vi "Get Channel Array Variables.vi"(8 "error in (no error)":errorcluster, 11 "LabVIEW Web Service Request":refnum<class "Web Request.lvclass">) -> (0 "error out":errorcluster, 3 "LabVIEW Web Service Request out":refnum<class "Web Request.lvclass">)   [LabVIEW 2018]
doc: "This VI sets all of the ESP variables for a single contact so it can be output from an ESP script."
uses:
  <vilib>/wsapi/Web Request.lvclass
  CAEN globals.vi
  <vilib>/wsapi/class/subVIs/Set Many String ESP Variables.vi
  <vilib>/wsapi/class/subVIs/Set Integer ESP Variable.vi
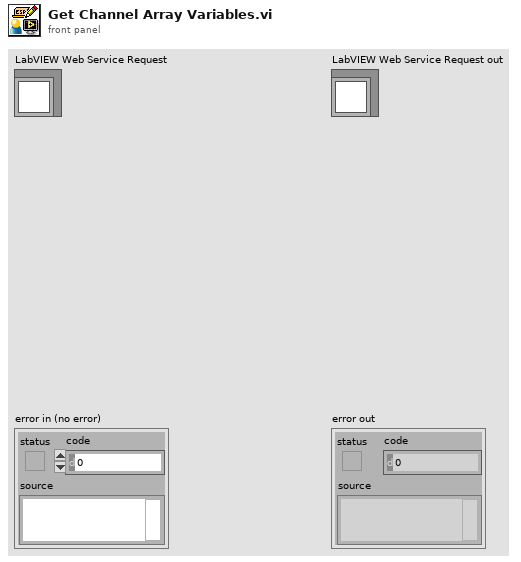
[diagram p1: front panel]
types:
  T1 = typedef "channel_cluster.ctl" = cluster{"Channel Name":string, "Crate":i32, "Card Type":string, "Card":i32, "Channel":i32, "Status Icon":picture, "Vmon (V)":dbl, "Vset (V)":dbl, "Imon (A)":dbl, "Iset (A)":dbl, "Timestamp":string, "ON/OFF":bool, "Status":string, "Vswmax (V)":dbl, "Flag":bool, "Vfile (V)":dbl, "Error Logged":bool[], "enable_file":bool}
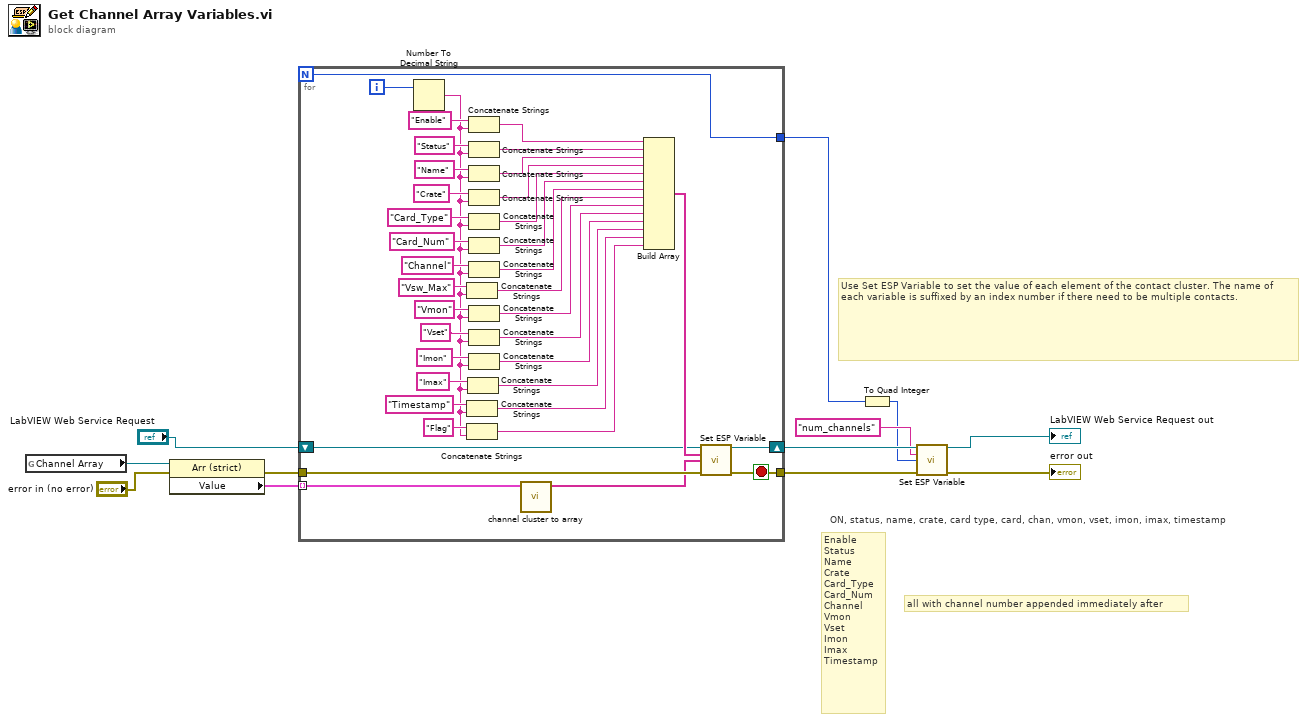
[diagram p0: block diagram]
diagram:
  # "all with channel number appended immediately after"
  # "Enable\nStatus\nName\nCrate\nCard_Type\nCard_Num\nChannel\nVmon\nVset\nImon\nImax\nTimestamp"
  # "ON, status, name, crate, card type, card, chan, vmon, vset, imon, imax, timestamp"
  # "Use Set ESP Variable to set the value of each element of the contact cluster. The name of each variable is suffixed by an index number if there need to be multiple contacts."
  n1 = global read "CAEN globals.vi" "Channel Array"() -> (w4:refnum<vi>)
  n2 = property class="Arr (strict)"(reference=w4, error in="error in (no error)") -> (error out=w1:errorcluster, "Value"=w3:T1[])  [unwired: 1 out]
  n3 = for {
    N -> [w21]
    tunnel: w3 -> [w20] mode=indexing
    tunnel: w1 -> [w50]
    tunnel: [w23] -> w11
    tunnel: [w21] -> w5
    shift-right: [w24] -> w10
    shift-left: "LabVIEW Web Service Request" -> [w31]
    i -> [w22]
    stop <- w23 stop-if-true
    n4 = Number To Decimal String(number=w22) -> (decimal integer string=w14:string)  [unwired: 1 in]
    n5 = Concatenate Strings("Vsw_Max" ("string"), w14) -> (w16:string)
    n6 = Concatenate Strings("Timestamp" ("string"), w14) -> (w26:string)
    n7 = Concatenate Strings("Flag" ("string"), w14) -> (w13:string)
    n8 = Concatenate Strings("Imax" ("string"), w14) -> (w27:string)
    n9 = Concatenate Strings("Enable" ("string"), w14) -> (w25:string)
    n10 = Concatenate Strings("Status" ("string"), w14) -> (w40:string)
    n11 = Concatenate Strings("Name" ("string"), w14) -> (w39:string)
    n12 = Concatenate Strings("Crate" ("string"), w14) -> (w38:string)
    n13 = Concatenate Strings("Card_Type" ("string"), w14) -> (w37:string)
    n14 = Concatenate Strings("Card_Num" ("string"), w14) -> (w36:string)
    n15 = Concatenate Strings("Channel" ("string"), w14) -> (w35:string)
    n16 = Concatenate Strings("Vmon" ("string"), w14) -> (w34:string)
    n17 = Concatenate Strings("Vset" ("string"), w14) -> (w33:string)
    n18 = Concatenate Strings("Imon" ("string"), w14) -> (w28:string)
    n19 = call "channel cluster to array.vi"("input cluster"=w20) -> ("Array"=w19:string[])  [unwired: 10 in]
    n20 = Build Array(w25, w40, w39, w38, w37, w36, w35, w16, w34, w33, w28, w27, w26, w13) -> (w32:string[])
    n21 = call-poly <vilib>:"Set ESP Variable.vi"("LabVIEW Web Service Request"=w31, "keys"=w32, "values"=w19, "error in (no error)"=w50) -> ("LabVIEW Web Service Request out"=w24:refnum<class "Web Request.lvclass">, "error out"=w23:errorcluster)  [unwired: 10 in]
  }
  n22 = To Quad Integer(1:w5) -> (0:w6:i64)
  n23 = call-poly <vilib>:"Set ESP Variable.vi"("LabVIEW Web Service Request"=w10, "key"="num_channels" ("string"), "value"=w6, "error in (no error)"=w11) -> ("LabVIEW Web Service Request out"=→"LabVIEW Web Service Request out":refnum<class "Web Request.lvclass">, "error out"=→"error out":errorcluster)  [unwired: 10 in]
